vi "load and linear filter.vi"() -> ()   [LabVIEW 2011]
uses:
  <userlib>/labvvis/New Image/New Image (Grey).vi
  <userlib>/labvvis/labvvis.lvlib
panel:
  in  "path to JPEG file":path
  out "Error":string
  in  "Mask":i8[][](array[numeric])=[[-1, -1, 0], [-1, 0, 1], [0, 1, 1]]
  out "new picture":picture
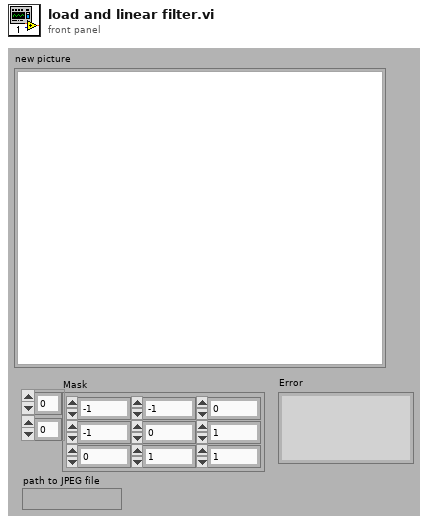
[diagram p1: front panel]
types:
  T1 = typedef "imagedata.ctl" = cluster{"image type":i32, "image depth":i32, "image":u8[], "mask":u8[], "colors":u32[], "Rectangle":cluster{"left":i16, "top":i16, "right":i16, "bottom":i16}}
  T2 = typedef "labvvis.lvlib/VVIS Image.ctl" = cluster{"Image ID":i16, "Channel ID":i16}
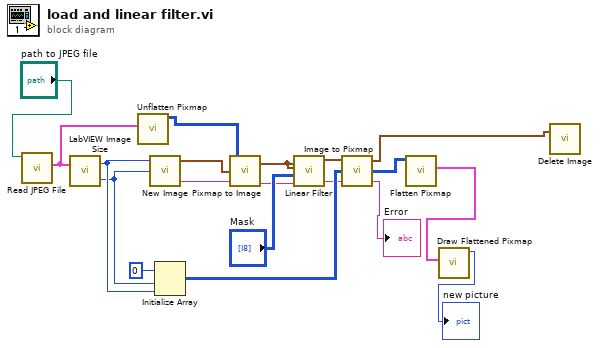
[diagram p0: block diagram]
diagram:
  n1 = call <vilib>:"Read JPEG File.vi"("path to JPEG file"="path to JPEG file") -> ("image data"=w11:T1)  [unwired: 8 in, 2 out]
  n2 = call <userlib>:"LabVIEW Image Size.vi"("Cluster"=w11) -> ("Width"=w14:i16, "Height"=w13:i16)
  n3 = call <vilib>:"Unflatten Pixmap.vi"("image data"=w11) -> ("24-bit pixmap"=w10:u32[][])  [unwired: 4 in, 6 out]
  n4 = call-poly <userlib>:"New Image.vi"("Height"=w13, "Width"=w14) -> ("Error"=w16:string, "VVIS Image"=w17:T2)  [unwired: 2 in]
  n5 = Initialize Array(0, w13, w14) -> (w18:i32[][])
  n6 = call <userlib>:"Pixmap to Image.vi"("Error"=w16, "Output Image"=w17, "Input Pixmap"=w10) -> ("Error"=w3:string, "Output Image"=w7:T2)
  n7 = call <userlib>:"Linear Filter.vi"("Error"=w3, "Mask"="Mask", "Output Image"=w7, "Input Image"=w7) -> ("Error"=w4:string, "Input Image"=w5:T2)  [unwired: 1 in, 1 out]
  n8 = call <userlib>:"Image to Pixmap.vi"("Error"=w4, "Output Pixmap"=w18, "Image"=w5) -> ("Error"=→"Error":string, "Output Pixmap"=w2:u32[][], "Image"=w15:T2)
  n9 = call <vilib>:"Flatten Pixmap.vi"("24-bit pixmap"=w2) -> ("image data"=w9:T1)  [unwired: 10 in]
  n10 = call <vilib>:"Draw Flattened Pixmap.vi"("image data"=w9) -> ("new picture"=→"new picture":picture)  [unwired: 8 in]
  n11 = call <userlib>:"Delete Image.vi"("Image"=w15) -> ()  [unwired: 2 in, 1 out]
